vi "Filter_test.vi"() -> ()   [LabVIEW 2024]
panel:
  out "x/y":dbl
  out "X 3":i64[](array[numeric])=[3500, 3500, 3500, 3500]
  out "X 2":dbl[](array[numeric])=[3500.0, 3500.0, 3500.0, 3500.0]
  out "x*2^n":i64=268435456 format="%.0d (x%x)"
  in  "kk":i64
  in  "pp":i64
  in  "bb":i64=276423
  in  "aa":i64
  in  "X":dbl[](array[numeric])=[3500.0, 3500.0, 3500.0, 3500.0]
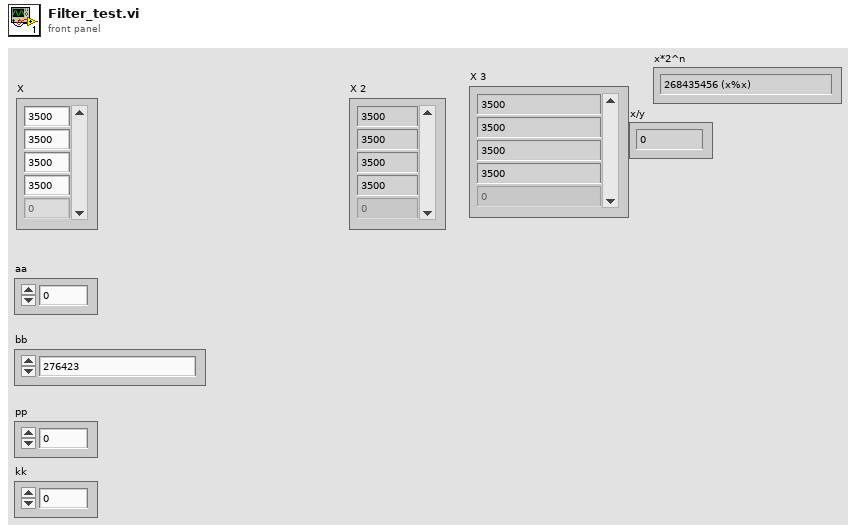
[diagram p1: front panel]
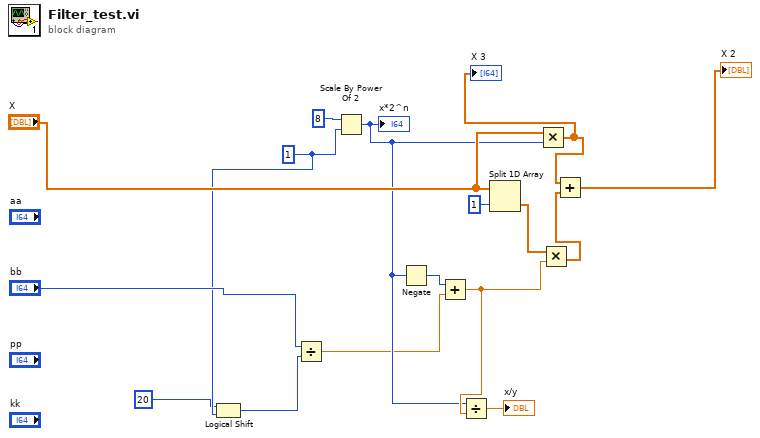
[diagram p0: block diagram]
diagram:
  w6 = i64 1
  n1 = Logical Shift(y=i16 20 ("n"), x=w6) -> (x << y=w4:i64)
  n2 = Divide(x="bb", y=w4) -> (x/y=w2:dbl)
  n3 = Scale By Power Of 2(n=i16 8, x=w6) -> (x*2^n=w3:i64)
  "x*2^n" <- w3
  n4 = Negate(x=w3) -> (-x=w15:i64)
  n5 = Add(x=w15, y=w2) -> (x+y=w9:dbl)
  n6 = Divide(x=w3, y=w9) -> (x/y=→"x/y":dbl)
  n7 = Split 1D Array(array="X", index=1) -> (second subarray=w13:dbl[])  [unwired: 1 out]
  n8 = Multiply(x="X", y=w3) -> (x*y=w10:dbl[])
  "X 3" <- w10
  n9 = Multiply(x=w13, y=w9) -> (x*y=w11:dbl[])
  n10 = Add(x=w10, y=w11) -> (x+y=→"X 2":dbl[])
